vi "Facade.vi"(0 "Data In":T4, 2 "Display State In":T2, 3 "Container State":T3) -> (6 "Data Out":T4, 7 "Display State Out":T2, 8 "Action":T1)   [LabVIEW 2019, in "Custom Calendar.xctl"]
uses:
  Custom Calendar.xctl
  Data Type.ctl
  <vilib>/_xctls/Container State.ctl
  State.ctl
  <vilib>/_xctls/Action.ctl
  <vilib>/_xctls/XControlSupport.lvlib
  <vilib>/Utility/miscctls.llb/LVRectTypeDef.ctl
panel:
  in  "stop":bool
  in  "LAST MONTH":bool
  out "Selected Date":string
  in  "NEXT MONTH":bool
  out "Month Name":string
  in  "Dates":string[][](table)
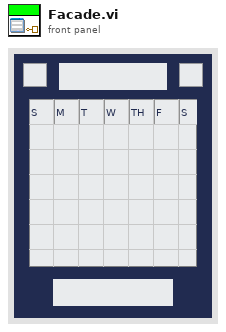
[diagram p1: front panel]
types:
  T1 = typedef "XControlSupport.lvlib/Action.ctl" = cluster{"Data Changed?":bool, "State Changed?":bool, "Action Name":string}
  T2 = typedef "Custom Calendar.xctl/State.ctl" = cluster{"Month":i32, "Day":i32, "Year":i32}
  T3 = typedef "XControlSupport.lvlib/Container State.ctl" = cluster{"Indicator?":bool, "Run Mode?":bool, " Refnum":refnum<vi>}
  T4 = typedef "Custom Calendar.xctl/Data Type.ctl" = string
  T5 = typedef "LVDateTimeRec.ctl" = cluster{"fractional second":dbl, "second":i32, "minute":i32, "hour":i32, "day of month":i32, "month":i32, "year":i32, "day of week":i32, "day of year":i32, "DST":i32}
  T6 = typedef "LVPoint32TypeDef.ctl" = cluster{"Horizontal":i32, "Vertical":i32}
  T7 = typedef "LVRectTypeDef.ctl" = cluster{"Left":i16, "Top":i16, "Right":i16, "Bottom":i16}
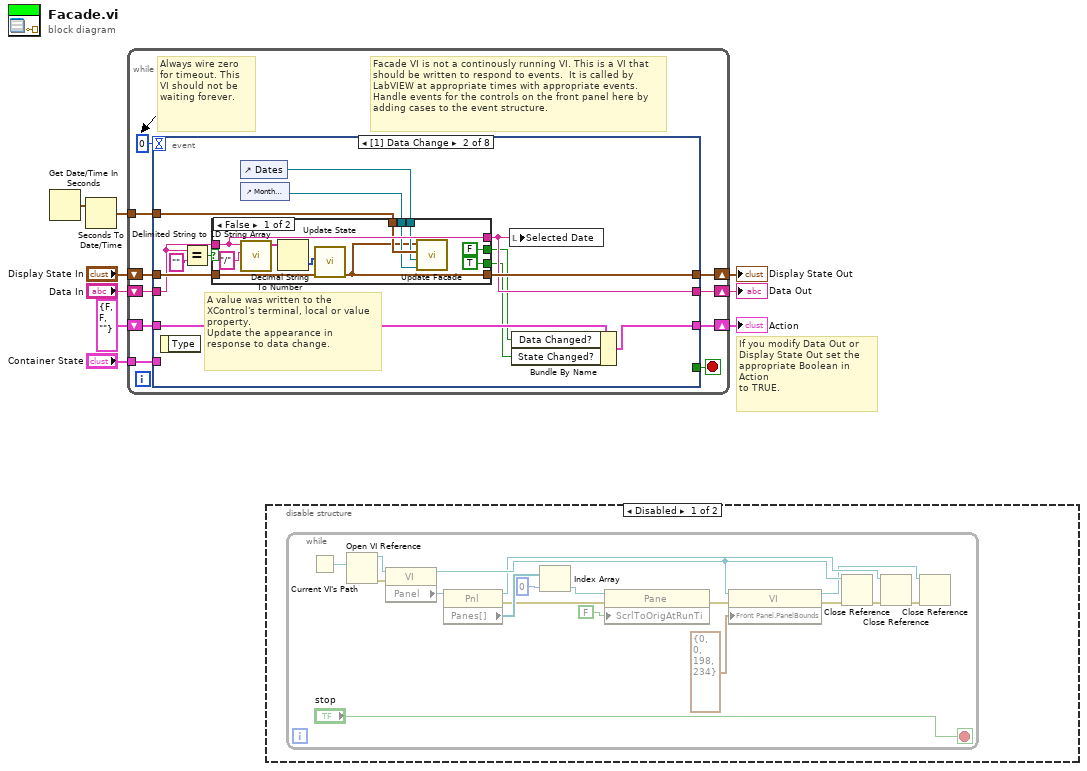
[diagram p0: block diagram]
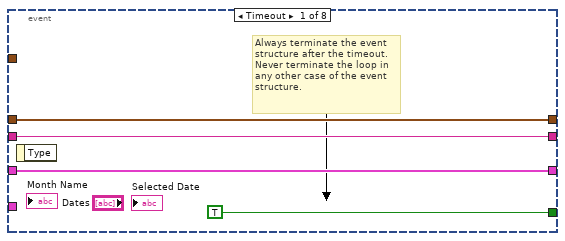
[diagram p3: hidden frame]
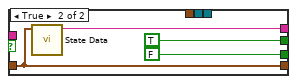
[diagram p4: hidden frame]
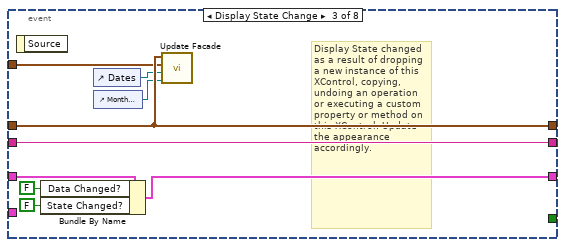
[diagram p5: hidden frame]
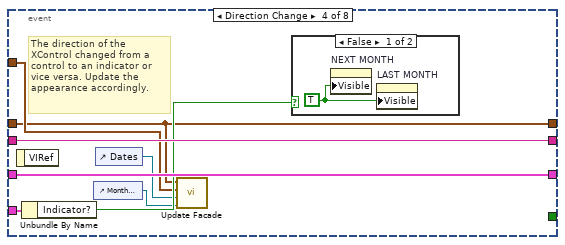
[diagram p6: hidden frame]
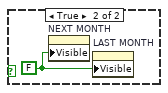
[diagram p7: hidden frame]
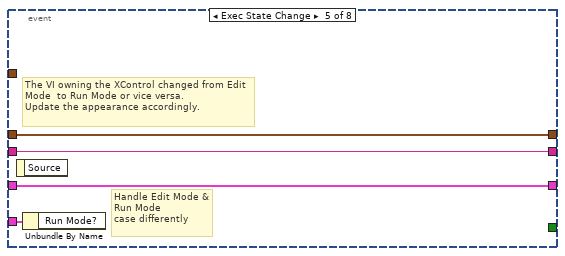
[diagram p8: hidden frame]
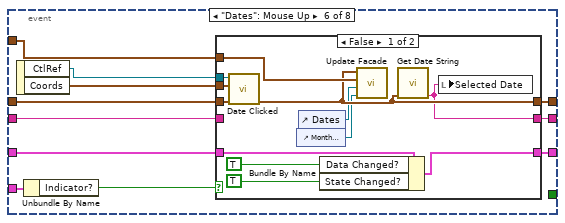
[diagram p9: hidden frame]
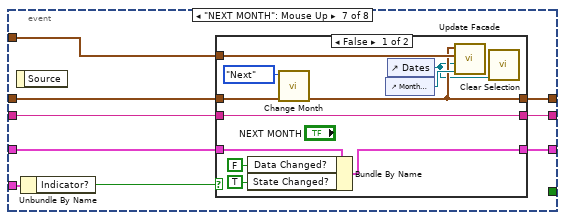
[diagram p11: hidden frame]
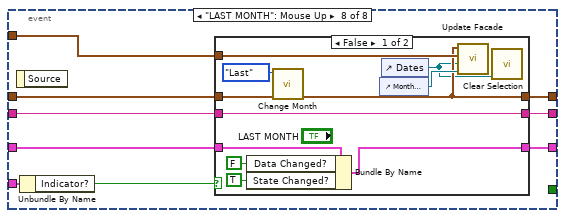
[diagram p13: hidden frame]
diagram:
  # "If you modify Data Out or\nDisplay State Out set the\nappropriate Boolean in Action\nto TRUE."
  n1 = Get Date/Time In Seconds() -> (seconds since 1Jan1904=w2:timestamp)
  n2 = Seconds To Date/Time(time stamp (now)=w2) -> (date time rec=w1:T5)  [unwired: 1 in]
  n3 = while {
    shift-right: [w18] -> w6
    shift-left: "Display State In" -> [w19]
    tunnel: "Container State" -> [w15]
    shift-right: [w13] -> w9
    shift-left: "Data In" -> [w14]
    shift-right: [w11] -> w4
    shift-left: T1 {"Data Changed?"=FALSE, "State Changed?"=FALSE, "Action Name"=""} ("Action") -> [w12]
    tunnel: w1 -> [w10]
    stop <- w17 stop-if-true
    # "Facade VI is not a continously running VI. This is a VI that should be written to respond to events.  It is called by LabVIEW at appropriate times with appropriate events. Handle events for the controls on the front panel here by adding cases to the event structure."
    # "Always wire zero for timeout. This\nVI should not be waiting forever."
    n4 = event shown="[1] Data Change" {
      selector: _ -> [_ _ _ _ _ _ _ _]
      dyn-events: _ -> [_ _ _ _ _ _ _ _]
      timeout: 0 -> [_ _ _ _ _ _ _ _]
      tunnel: w19 -> [w21 w34 w55 w63 w73 w85 w109 w132]
      tunnel: [w21 w33 w55 w63 w73 w84 w103 w126] -> w18
      tunnel: [TRUE _ _ _ _ _ _ _] -> w17
      tunnel: w15 -> [_ _ _ w68 w74 w79 w105 w128]
      tunnel: w14 -> [w20 w32 w56 w67 w72 w82 w102 w125]
      tunnel: [w20 w29 w56 w67 w72 w80 w106 w129] -> w13
      tunnel: [w22 w35 w59 w66 w71 w81 w107 w130] -> w11
      tunnel: w12 -> [w22 w36 w60 w66 w71 w83 w108 w131]
      tunnel: w10 -> [_ w26 w54 w64 _ w75 w101 w124]
      event Timeout {
        # "Always terminate the event\nstructure after the timeout. Never terminate the loop in any other case of the event structure."
        n5 = event-data() -> ()  [unwired: 1 in, 1 out]
      }
      event Data Change {
        # "A value was written to the XControl's terminal, local or value property.\nUpdate the appearance in response to data change."
        n6 = event-data() -> ()  [unwired: 1 in, 1 out]
        n7 = Equal?(x=w32, y="") -> (x = y?=w30:bool)
        n8 = control-ref of="Dates"() -> (w25:refnum<vi>)
        n9 = control-ref of="Month Name"() -> (w24:refnum<vi>)
        n10 = case shown="False" w30 {
          tunnel: w34 -> [w45 w51]
          tunnel: [w37 w51] -> w33
          tunnel: w32 -> [w43 _]
          tunnel: [w43 w50] -> w29
          tunnel: [TRUE FALSE] -> w28
          tunnel: [FALSE TRUE] -> w27
          tunnel: w26 -> [w40 _]
          tunnel: w25 -> [w39 _]
          tunnel: w24 -> [w38 _]
          frame False {
            n11 = call <vilib>:"Delimited String to 1D String Array.vi"("delimiter"="/", "delimited string"=w43) -> ("string array"=w46:string[])  [unwired: 9 in]
            n12 = Decimal String To Number(string=w46) -> (number=w44:i32[])  [unwired: 2 in, 1 out]
            n13 = call "Update State.vi"("Display State In"=w45, "Data In"=w44) -> ("Display State Out"=w37:cluster{"Month":i32, "Day":i32, "Year":i32})  [unwired: 9 in]
            n14 = call "Update Facade.vi"("Month Name"=w38, "Dates"=w39, "date time rec"=w40, "Display State In"=w37) -> ()  [unwired: 8 in]
          }
          frame True {
            n15 = call "State Data.vi"("Display State In"=w51) -> ("Data Out"=w50:string)  [unwired: 10 in]
          }
        }
        n16 = local write "Selected Date"(w29) -> ()
        n17 = Bundle By Name(cluster=w36, "Data Changed?"=w27, "State Changed?"=w28) -> (w35:T1)
      }
      event Display State Change {
        # "Display State changed as a result of dropping a new instance of this XControl, copying, undoing an operation or executing a custom property or method on this XControl. Update the appearance accordingly."
        n18 = event-data() -> ()  [unwired: 1 in, 1 out]
        n19 = Bundle By Name(cluster=w60, "Data Changed?"=FALSE, "State Changed?"=FALSE) -> (w59:T1)
        n20 = control-ref of="Dates"() -> (w52:refnum<vi>)
        n21 = control-ref of="Month Name"() -> (w53:refnum<vi>)
        n22 = call "Update Facade.vi"("Month Name"=w53, "Dates"=w52, "date time rec"=w54, "Display State In"=w55) -> ()  [unwired: 8 in]
      }
      event Direction Change {
        # "The direction of the XControl changed from a control to an indicator or vice versa. Update the appearance accordingly."
        n23 = event-data() -> ()  [unwired: 1 in, 1 out]
        n24 = Unbundle By Name(w68) -> ("Indicator?"=w65:bool)
        n25 = control-ref of="Month Name"() -> (w61:refnum<vi>)
        n26 = control-ref of="Dates"() -> (w62:refnum<vi>)
        n27 = call "Update Facade.vi"("Month Name"=w61, "Dates"=w62, "date time rec"=w64, "Display State In"=w63) -> ()  [unwired: 8 in]
        n28 = case shown="False" w65 {
          frame False {
            w69 = TRUE ("Visible")
            n29 = property on="NEXT MONTH" class="Bool (strict)"("Visible"=w69) -> ()  [unwired: 2 in, 2 out]
            n30 = property on="LAST MONTH" class="Bool (strict)"("Visible"=w69) -> ()  [unwired: 2 in, 2 out]
          }
          frame True {
            w70 = FALSE ("Visible")
            n31 = property on="NEXT MONTH" class="Bool (strict)"("Visible"=w70) -> ()  [unwired: 2 in, 2 out]
            n32 = property on="LAST MONTH" class="Bool (strict)"("Visible"=w70) -> ()  [unwired: 2 in, 2 out]
          }
        }
      }
      event Exec State Change {
        # "The VI owning the XControl changed from Edit Mode  to Run Mode or vice versa.\nUpdate the appearance accordingly."
        # "Handle Edit Mode & Run Mode\ncase differently"
        n33 = event-data() -> ()  [unwired: 1 in, 1 out]
        n34 = Unbundle By Name(w74) -> ()  [unwired: 1 out]
      }
      event "Dates": Mouse Up {
        n35 = event-data() -> ("CtlRef"=w77:refnum<vi>, "Coords"=w76:T6)  [unwired: 1 in]
        n36 = Unbundle By Name(w79) -> ("Indicator?"=w78:bool)
        n37 = case shown="False" w78 {
          tunnel: w85 -> [w97 w100]
          tunnel: [w89 w100] -> w84
          tunnel: w83 -> [w96 w98]
          tunnel: w82 -> [_ w99]
          tunnel: [w93 w98] -> w81
          tunnel: [w88 w99] -> w80
          tunnel: w77 -> [w92 _]
          tunnel: w76 -> [w91 _]
          tunnel: w75 -> [w90 _]
          frame False {
            n38 = call "Date Clicked.vi"("Display State In"=w97, "Coords"=w91, "Dates"=w92) -> ("Display State Out"=w89:cluster{"Month":i32, "Day":i32, "Year":i32})  [unwired: 8 in]
            n39 = control-ref of="Month Name"() -> (w86:refnum<vi>)
            n40 = control-ref of="Dates"() -> (w87:refnum<vi>)
            n41 = Bundle By Name(cluster=w96, "Data Changed?"=TRUE, "State Changed?"=TRUE) -> (w93:T1)
            n42 = call "Update Facade.vi"("Month Name"=w86, "Dates"=w87, "date time rec"=w90, "Display State In"=w89) -> ()  [unwired: 8 in]
            n43 = call "Get Date String.vi"("Display State In"=w89) -> ("Date String Out"=w88:string)  [unwired: 10 in]
            n44 = local write "Selected Date"(w88) -> ()
          }
          frame True {
          }
        }
      }
      event "NEXT MONTH": Mouse Up {
        n45 = event-data() -> ()  [unwired: 1 in, 1 out]
        n46 = Unbundle By Name(w105) -> ("Indicator?"=w104:bool)
        n47 = case shown="False" w104 {
          tunnel: w109 -> [w113 w123]
          tunnel: w108 -> [w120 w122]
          tunnel: [w117 w122] -> w107
          tunnel: [w116 w121] -> w106
          tunnel: [w112 w123] -> w103
          tunnel: w102 -> [w116 w121]
          tunnel: w101 -> [w115 _]
          frame False {
            n48 = Bundle By Name(cluster=w120, "Data Changed?"=FALSE, "State Changed?"=TRUE) -> (w117:T1)
            n49 = call "Change Month.vi"("Display State In"=w113, "Change"=enum16{"Next", "Last"}."Next") -> ("Display State Out"=w112:cluster{"Month":i32, "Day":i32, "Year":i32})  [unwired: 9 in]
            n50 = control-ref of="Month Name"() -> (w114:refnum<vi>)
            n51 = control-ref of="Dates"() -> (w110:refnum<vi>)
            n52 = call "Update Facade.vi"("Month Name"=w114, "Dates"=w110, "date time rec"=w115, "Display State In"=w112) -> ()  [unwired: 8 in]
            n53 = call "Clear Selection.vi"("Dates In"=w110) -> ()  [unwired: 11 in]
          }
          frame True {
          }
        }
      }
      event "LAST MONTH": Mouse Up {
        n54 = event-data() -> ()  [unwired: 1 in, 1 out]
        n55 = Unbundle By Name(w128) -> ("Indicator?"=w127:bool)
        n56 = case shown="False" w127 {
          tunnel: w132 -> [w136 w144]
          tunnel: w131 -> [w143 w146]
          tunnel: [w140 w146] -> w130
          tunnel: [w139 w145] -> w129
          tunnel: [w135 w144] -> w126
          tunnel: w125 -> [w139 w145]
          tunnel: w124 -> [w138 _]
          frame False {
            n57 = Bundle By Name(cluster=w143, "Data Changed?"=FALSE, "State Changed?"=TRUE) -> (w140:T1)
            n58 = call "Change Month.vi"("Display State In"=w136, "Change"=enum16{"Next", "Last"}."Last") -> ("Display State Out"=w135:cluster{"Month":i32, "Day":i32, "Year":i32})  [unwired: 9 in]
            n59 = control-ref of="Month Name"() -> (w137:refnum<vi>)
            n60 = control-ref of="Dates"() -> (w133:refnum<vi>)
            n61 = call "Update Facade.vi"("Month Name"=w137, "Dates"=w133, "date time rec"=w138, "Display State In"=w135) -> ()  [unwired: 8 in]
            n62 = call "Clear Selection.vi"("Dates In"=w133) -> ()  [unwired: 11 in]
          }
          frame True {
          }
        }
      }
    }
  }
  "Display State Out" <- w6
  "Data Out" <- w9
  "Action" <- w4
  n63 = disable-structure shown="Disabled" {
    frame Disabled {
      n64 = while {
        stop <- "stop" stop-if-true
        n65 = Current VI's Path() -> (path=w163:path)
        n66 = Open VI Reference(vi path=w163) -> (vi reference=w162:refnum<vi>, error out=w161:errorcluster)  [unwired: 5 in]
        n67 = property class="VI"(reference=w162, error in=w161) -> (reference out=w152:refnum<vi>, "Panel"=w160:refnum<vi>)  [unwired: 1 out]
        n68 = property class="Pnl"(reference=w160) -> (reference out=w150:refnum<vi>, error out=w155:errorcluster, "Panes[]"=w159:refnum<vi>[])  [unwired: 1 in]
        n69 = Index Array(array=w159, index=0) -> (element=w157:refnum<vi>)
        n70 = property class="Pane"(reference=w157, error in=w155, "ScrlToOrigAtRunTi"=FALSE ("Scroll To Origin At Run Time")) -> (error out=w154:errorcluster)  [unwired: 1 out]
        n71 = property class="VI"(reference=w152, error in=w154, "Front Panel.PanelBounds"=T7 {"Left"=0, "Top"=0, "Right"=198, "Bottom"=234} ("Front Panel Window:Panel Bounds")) -> (reference out=w148:refnum<vi>, error out=w151:errorcluster)
        n72 = Close Reference(reference=w152, error in (no error)=w151) -> (error out=w149:errorcluster)
        n73 = Close Reference(reference=w150, error in (no error)=w149) -> (error out=w147:errorcluster)
        n74 = Close Reference(reference=w148, error in (no error)=w147) -> ()  [unwired: 1 out]
      }
    }
    frame Enabled {
    }
  }
